vi "run.vi"(8 "error in (no error)":errorcluster, 11 "IntrinsicImagingMG091001 in":refnum<class "DataCollectionMG091001IntrinsicImaging.lvclass">) -> (0 "error out":errorcluster, 3 "IntrinsicImagingMG091001 out":refnum<class "DataCollectionMG091001IntrinsicImaging.lvclass">)   [LabVIEW 2010, in "DataCollectionMG091001IntrinsicImaging.lvclass"]
uses:
  DataCollectionMG091001IntrinsicImaging.lvclass
  sweep_part_enum.ctl
  average_save_type_enum.ctl
  individual_sweeps_saving_enum.ctl
  main/labview_source/controls/undock_button.ctl
  DataCollectionMG091001IntrinsicImaging.lvclass/DataCollectionMG091001IntrinsicImaging.ctl
  DataCollectionDL091104Scaffold/DataCollectionDL091104Scaffold/DataCollectionDL091104Scaffold.lvclass
  common/classes/ErrorController/ErrorController/class_data.vi
  GenericDataCollection/GenericDataCollection/GenericDataCollection.lvclass
  common/classes/ErrorController/ErrorController/ErrorController.lvclass
panel:
  in  "button:undock":T1
  in  "Tab Control":enum32{"User", "About"}(tab)
  in  "Sweep":i32(slide) scale=1.0..1.1
  in  "average over time":bool
  in  "Average over sweeps?":bool
  in  "average save type enum":T2 caption="What to save..."
  in  "include sweep?":bool
  in  "Time":dbl[unit](slide) min=0.0 scale=0.0..1.0
  in  "sweep part":T3
  in  "overlay button":bool
  in  "save control?":bool
  in  "How to save individual sweeps:":T4
  in  "finished?":bool
  # "Browse data"
  # "Saving parameters"
  # "DataCollectionMG091001IntrinsicImaging\n\nImplemented by:\nMaurice Göldi, University of Zürich, Switezrland"
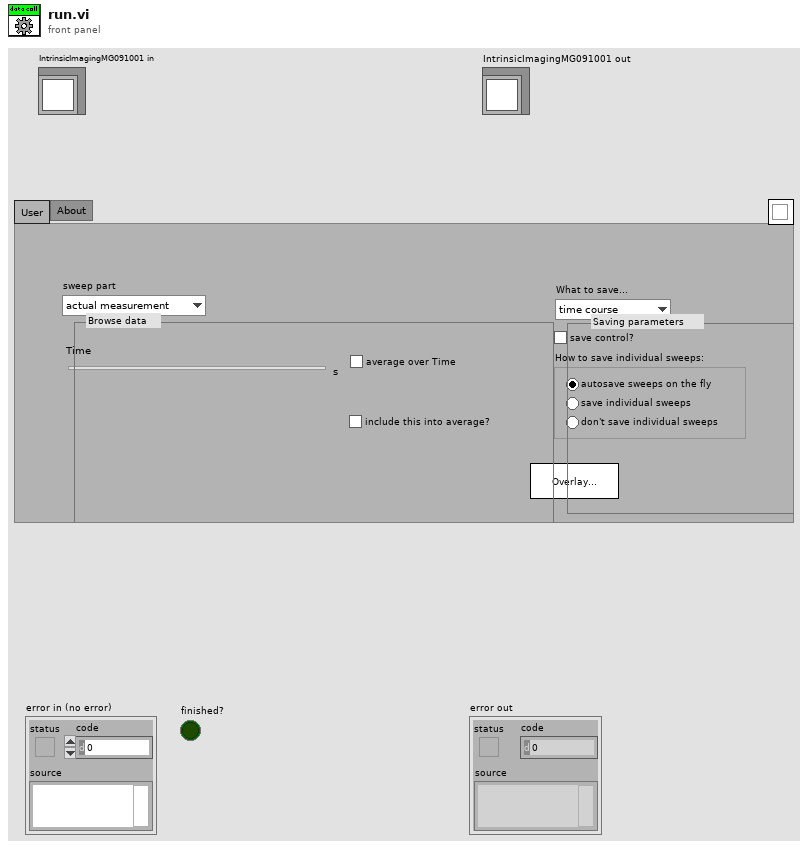
[diagram p1: front panel]
types:
  T1 = typedef "undock_button.ctl" = bool
  T2 = typedef "DataCollectionMG091001IntrinsicImaging.lvclass/average_save_type_enum.ctl" = enum16{"time course", "time average", "time course and average"}
  T3 = typedef "DataCollectionMG091001IntrinsicImaging.lvclass/sweep_part_enum.ctl" = enum16{"actual measurement", "control"}
  T4 = typedef "DataCollectionMG091001IntrinsicImaging.lvclass/individual_sweeps_saving_enum.ctl" = enum32{"autosave sweeps on the fly", "save individual sweeps", "don't save individual sweeps"}
  T5 = enum8{"Enabled", "Disabled", "Disabled and Grayed Out"}
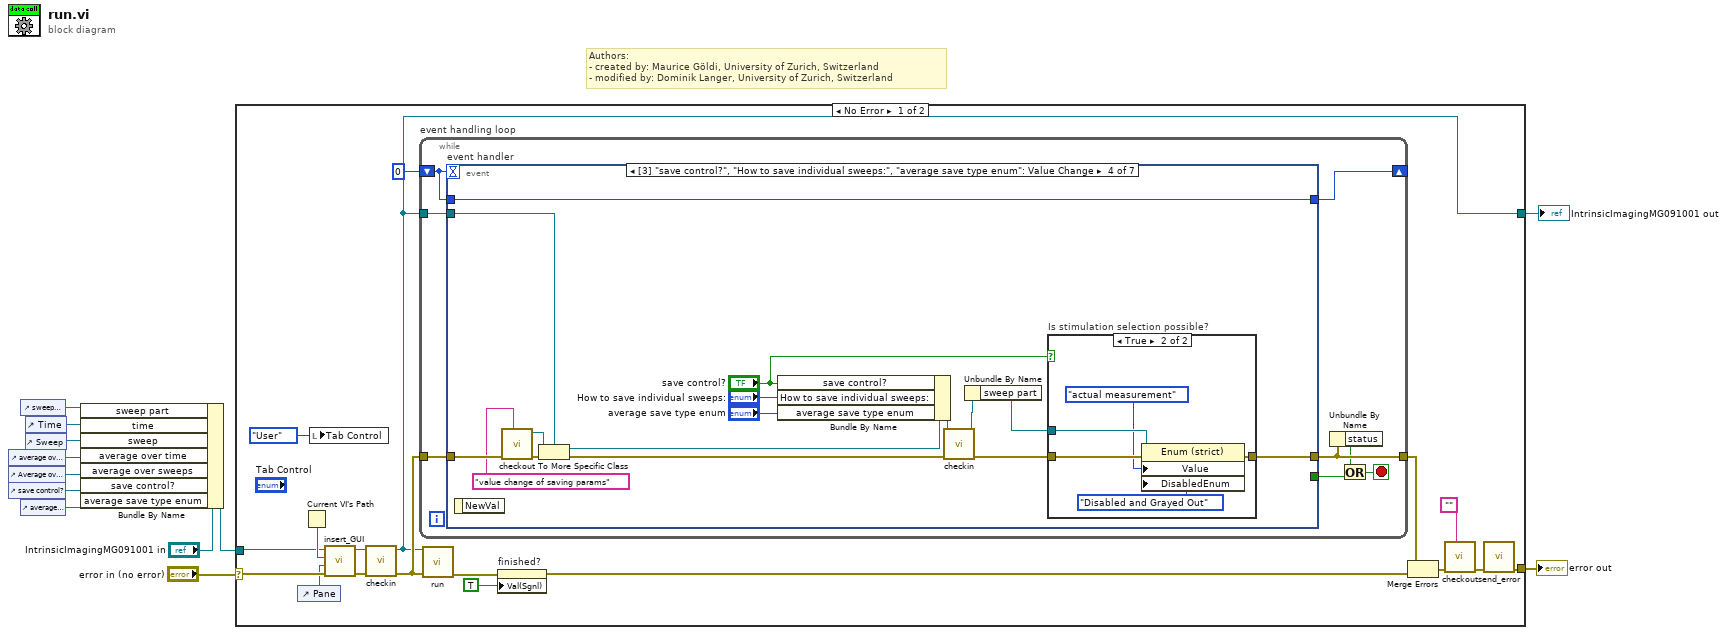
[diagram p0: block diagram]
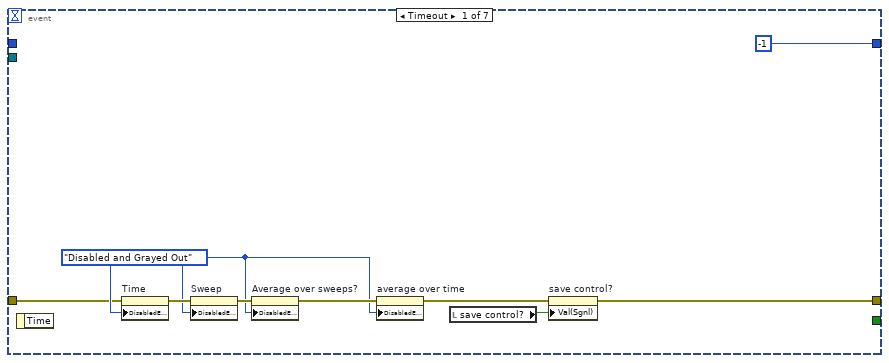
[diagram p2: hidden frame]
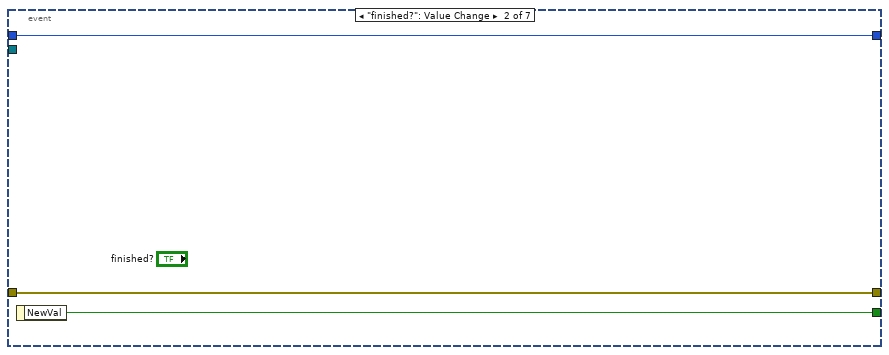
[diagram p3: hidden frame]
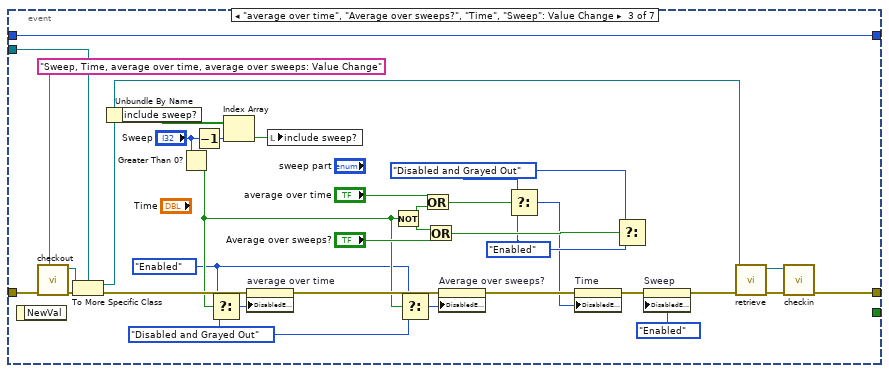
[diagram p4: hidden frame]
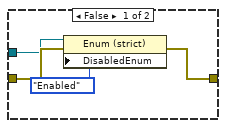
[diagram p5: hidden frame]
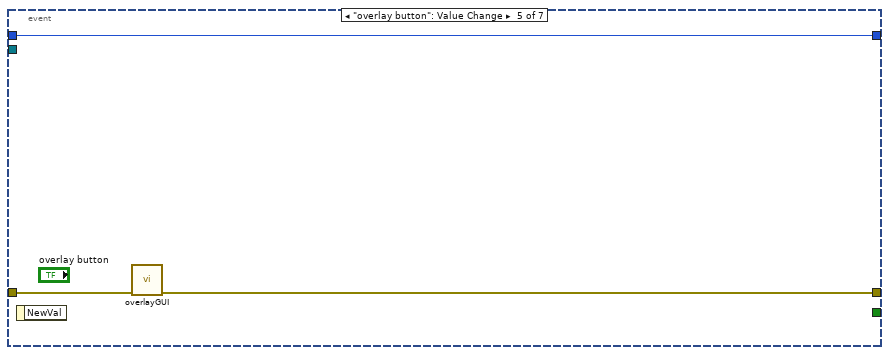
[diagram p6: hidden frame]
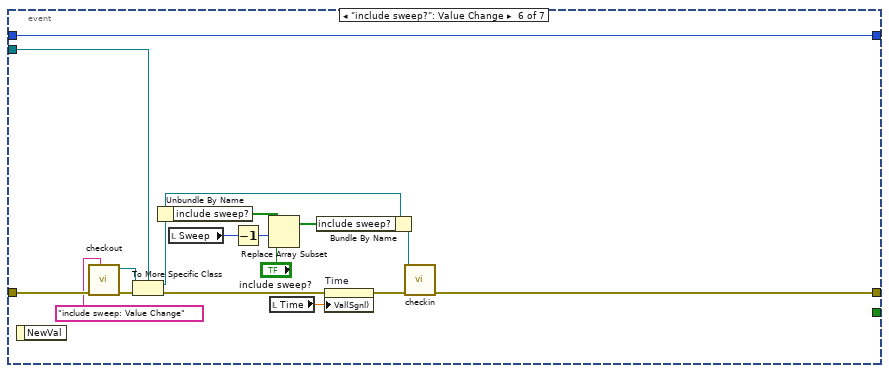
[diagram p7: hidden frame]
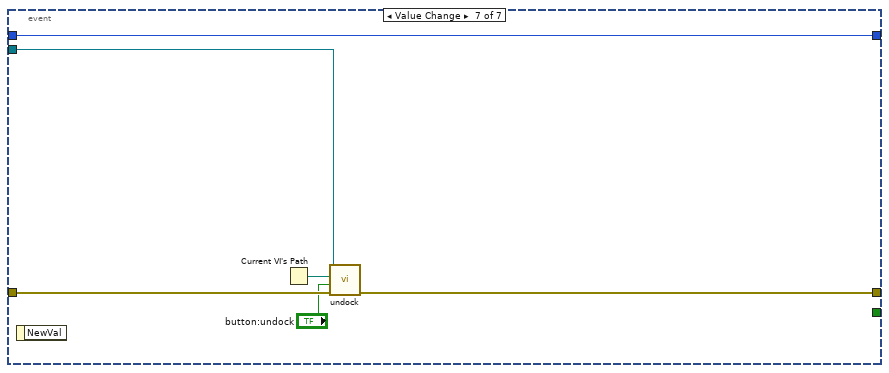
[diagram p8: hidden frame]
diagram:
  # "Authors: \n- created by: Maurice Göldi, University of Zurich, Switzerland\n- modified by: Dominik Langer, University of Zurich, Switzerland"
  n1 = control-ref of="average over time"() -> (w7:refnum<vi>)
  n2 = control-ref of="Average over sweeps?"() -> (w8:refnum<vi>)
  n3 = control-ref of="save control?"() -> (w4:refnum<vi>)
  n4 = control-ref of="sweep part"() -> (w1:refnum<vi>)
  n5 = control-ref of="average save type enum"() -> (w3:refnum<vi>)
  n6 = control-ref of="Time"() -> (w2:refnum<vi>)
  n7 = control-ref of="Sweep"() -> (w9:refnum<vi>)
  n8 = Bundle By Name(cluster="IntrinsicImagingMG091001 in", "sweep part"=w1, "time"=w2, "sweep"=w9, "average over time"=w7, "average over sweeps"=w8, "save control?"=w4, "average save type enum"=w3) -> (w5:refnum<class "DataCollectionMG091001IntrinsicImaging.lvclass">)
  n9 = case shown="No Error" "error in (no error)" {
    selector: "error in (no error)" -> [w21 w135]
    tunnel: [w17 w135] -> w12
    tunnel: [w15 w136] -> w11
    tunnel: w5 -> [w20 w136]
    frame No Error {
      n10 = control-ref of="Pane"() -> (w19:refnum<vi>)
      n11 = Current VI's Path() -> (path=w22:path)
      n12 = local write "Tab Control"(enum32{"User", "About"}."User" ("Tab Control")) -> ()
      n13 = call-dynamic "insert_GUI.vi"("error in (no error)"=w21, "Pane"=w19, "VI path"=w22, "GenericComponent in"=w20) -> ("error out"=w13:errorcluster, "GenericComponent out"=w14:refnum<class "DataCollectionMG091001IntrinsicImaging.lvclass">)  [unwired: 6 in]
      n14 = call-dynamic "checkin.vi"("error in (no error)"=w13, "GenericDataCollection in"=w14) -> ("error out"=w27:errorcluster, "GenericDataCollection out"=w15:refnum<class "DataCollectionMG091001IntrinsicImaging.lvclass">)  [unwired: 8 in]
      n15 = while "event handling loop" {
        shift-right: [w36] -> _
        shift-left: 0 -> [w35]
        tunnel: w27 -> [w38]
        tunnel: [w33] -> w26
        tunnel: w15 -> [w37]
        stop <- w31 stop-if-true
        n16 = event "event handler" shown="[3] \"save control?\", \"How to save individual sweeps:\", \"average save type enum\": Value Change" {
          selector: _ -> [_ _ _ _ _ _ _]
          dyn-events: _ -> [_ _ _ _ _ _ _]
          timeout: w35 -> [_ _ _ _ _ _ _]
          tunnel: [w40 w49 w81 w87 w109 w112 w131] -> w33
          tunnel: w38 -> [w39 w49 w82 w95 w110 w117 w132]
          tunnel: w37 -> [_ _ w78 w96 _ w120 w133]
          tunnel: [-1 w50 w83 w99 w111 w128 w134] -> w36
          tunnel: w35 -> [_ w50 w83 w99 w111 w128 w134]
          tunnel: [_ w48 _ _ _ _ _] -> w34
          event Timeout {
            w43 = T5."Disabled and Grayed Out" ("Disabled")
            n17 = event-data() -> ()  [unwired: 1 in, 1 out]
            n18 = property on="Time" class="Slide (strict)"(error in=w39, "DisabledEnum"=w43) -> (error out=w44:errorcluster)  [unwired: 1 in, 1 out]
            n19 = property on="Sweep" class="Slide (strict)"(error in=w44, "DisabledEnum"=w43) -> (error out=w45:errorcluster)  [unwired: 1 in, 1 out]
            n20 = property on="Average over sweeps?" class="Bool (strict)"(error in=w45, "DisabledEnum"=w43) -> (error out=w46:errorcluster)  [unwired: 1 in, 1 out]
            n21 = property on="average over time" class="Bool (strict)"(error in=w46, "DisabledEnum"=w43) -> (error out=w41:errorcluster)  [unwired: 1 in, 1 out]
            n22 = local read "save control?"() -> (w42:bool)
            n23 = property on="save control?" class="Bool (strict)"(error in=w41, "Val(Sgnl)"=w42) -> (error out=w40:errorcluster)  [unwired: 1 in, 1 out]
          }
          event "finished?": Value Change {
            n24 = event-data() -> ("NewVal"=w48:bool)  [unwired: 1 in]
          }
          event "average over time", "Average over sweeps?", "Time", "Sweep": Value Change {
            w59 = T5."Disabled and Grayed Out" ("Disabled")
            w58 = T5."Enabled" ("Disabled")
            w62 = T5."Disabled and Grayed Out" ("f")
            w61 = T5."Enabled" ("Disabled")
            n25 = event-data() -> ()  [unwired: 1 in, 1 out]
            n26 = call "checkout.vi"("locked by?"="Sweep, Time, average over time, average over sweeps: Value Change", "error in (no error)"=w82) -> ("error out"=w80:errorcluster, "GenericDataCollection out"=w79:refnum<class "GenericDataCollection.lvclass">)  [unwired: 8 in]
            n27 = To More Specific Class(target class=w78, reference=w79, error in=w80) -> (specific class reference=w52:refnum<class "DataCollectionMG091001IntrinsicImaging.lvclass">, error out=w68:errorcluster)
            n28 = Unbundle By Name(w52) -> ("include sweep?"=w76:bool[])
            n29 = Greater Than 0?(x="Sweep") -> (x > 0?=w64:bool)
            n30 = Decrement(x="Sweep") -> (x-1=w74:i32)
            n31 = Select(t=w61, s=w64, f=w62) -> (s? t:f=w67:T5)
            n32 = Index Array(array=w76, index=w74) -> (element=w75:bool)
            n33 = property on="average over time" class="Bool (strict)"(error in=w68, "DisabledEnum"=w67) -> (error out=w72:errorcluster)  [unwired: 1 in, 1 out]
            n34 = local write "include sweep?"(w75) -> ()
            n35 = Not(x=w64) -> (.not. x?=w70:bool)
            n36 = Select(t=w61, s=w64, f=w62) -> (s? t:f=w63:T5)
            n37 = Or(x="average over time", y=w70) -> (x .or. y?=w60:bool)
            n38 = Or(x=w70, y="Average over sweeps?") -> (x .or. y?=w65:bool)
            n39 = property on="Average over sweeps?" class="Bool (strict)"(error in=w72, "DisabledEnum"=w63) -> (error out=w69:errorcluster)  [unwired: 1 in, 1 out]
            n40 = Select(t=w59, s=w60, f=w58) -> (s? t:f=w57:T5)
            n41 = property on="Time" class="Slide (strict)"(error in=w69, "DisabledEnum"=w57) -> (error out=w55:errorcluster)  [unwired: 1 in, 1 out]
            n42 = Select(t=w59, s=w65, f=w58) -> ()  [unwired: 1 out]
            n43 = property on="Sweep" class="Slide (strict)"(error in=w55, "DisabledEnum"=T5."Enabled" ("Disabled")) -> (error out=w54:errorcluster)  [unwired: 1 in, 1 out]
            n44 = call-dynamic "retrieve.vi"("error in (no error)"=w54, "DL090215DataCollection in"=w52) -> ("error out"=w53:errorcluster, "DL090215DataCollection out"=w51:refnum<class "DataCollectionMG091001IntrinsicImaging.lvclass">)  [unwired: 8 in]
            n45 = call-dynamic "checkin.vi"("error in (no error)"=w53, "GenericDataCollection in"=w51) -> ("error out"=w81:errorcluster)  [unwired: 8 in, 1 out]
          }
          event "save control?": Value Change {
            n46 = event-data() -> ()  [unwired: 1 in, 1 out]
            n47 = call "checkout.vi"("locked by?"="value change of saving params", "error in (no error)"=w95) -> ("error out"=w94:errorcluster, "GenericDataCollection out"=w93:refnum<class "GenericDataCollection.lvclass">)  [unwired: 8 in]
            n48 = To More Specific Class(target class=w96, reference=w93, error in=w94) -> (specific class reference=w92:refnum<class "DataCollectionMG091001IntrinsicImaging.lvclass">, error out=w90:errorcluster)
            n49 = Bundle By Name(cluster=w92, "save control?"="save control?", "How to save individual sweeps:"="How to save individual sweeps:", "average save type enum"="average save type enum") -> (w91:refnum<class "DataCollectionMG091001IntrinsicImaging.lvclass">)
            n50 = call-dynamic "checkin.vi"("error in (no error)"=w90, "GenericDataCollection in"=w91) -> ("error out"=w88:errorcluster, "GenericDataCollection out"=w86:refnum<class "DataCollectionMG091001IntrinsicImaging.lvclass">)  [unwired: 8 in]
            n51 = Unbundle By Name(w86) -> ("sweep part"=w85:refnum<vi>)
            n52 = case "Is stimulation selection possible?" shown="True" "save control?" {
              tunnel: w88 -> [w103 w108]
              tunnel: [w102 w107] -> w87
              tunnel: w85 -> [w101 w106]
              frame False {
                n53 = property class="Enum (strict)"(reference=w101, error in=w103, "DisabledEnum"=T5."Enabled" ("Disabled")) -> (error out=w102:errorcluster)  [unwired: 1 out]
              }
              frame True {
                n54 = property class="Enum (strict)"(reference=w106, error in=w108, "Value"=enum16{"actual measurement", "control"}."actual measurement", "DisabledEnum"=T5."Disabled and Grayed Out" ("Disabled")) -> (error out=w107:errorcluster)  [unwired: 1 out]
              }
            }
          }
          event "overlay button": Value Change {
            n55 = event-data() -> ()  [unwired: 1 in, 1 out]
            n56 = call "overlayGUI.vi"("error in (no error)"=w110) -> ("error out"=w109:errorcluster)  [unwired: 10 in]
          }
          event "include sweep?": Value Change {
            n57 = event-data() -> ()  [unwired: 1 in, 1 out]
            n58 = call "checkout.vi"("locked by?"="include sweep: Value Change", "error in (no error)"=w117) -> ("error out"=w122:errorcluster, "GenericDataCollection out"=w121:refnum<class "GenericDataCollection.lvclass">)  [unwired: 8 in]
            n59 = To More Specific Class(target class=w120, reference=w121, error in=w122) -> (specific class reference=w119:refnum<class "DataCollectionMG091001IntrinsicImaging.lvclass">, error out=w114:errorcluster)
            n60 = Unbundle By Name(w119) -> ("include sweep?"=w126:bool[])
            n61 = local read "Sweep"() -> (w123:i32)
            n62 = Decrement(x=w123) -> (x-1=w124:i32)
            n63 = Replace Array Subset(array=w126, new element="include sweep?", index=w124) -> (w125:bool[])
            n64 = local read "Time"() -> (w115:dbl[unit])
            n65 = Bundle By Name(cluster=w119, "include sweep?"=w125) -> (w118:refnum<class "DataCollectionMG091001IntrinsicImaging.lvclass">)
            n66 = property on="Time" class="Slide (strict)"(error in=w114, "Val(Sgnl)"=w115) -> (error out=w113:errorcluster)  [unwired: 1 in, 1 out]
            n67 = call-dynamic "checkin.vi"("error in (no error)"=w113, "GenericDataCollection in"=w118) -> ("error out"=w112:errorcluster)  [unwired: 8 in, 1 out]
          }
          event Value Change {
            n68 = event-data() -> ()  [unwired: 1 in, 1 out]
            n69 = Current VI's Path() -> (path=w129:path)
            n70 = call-dynamic "undock.vi"("error in (no error)"=w132, "undock?"="button:undock", "VI path"=w129, "GenericComponent in"=w133) -> ("error out"=w131:errorcluster)  [unwired: 6 in, 1 out]
          }
        }
        n71 = Unbundle By Name(w33) -> ("status"=w32:bool)
        n72 = Or(x=w32, y=w34) -> (x .or. y?=w31:bool)
      }
      n73 = call-parent "run.vi"("error in (no error)"=w27, "DataCollectionDL091104Scaffold.lvclass out"=w15) -> ("error out"=w30:errorcluster)  [unwired: 8 in, 1 out]
      n74 = property on="finished?" class="Bool (strict)"(error in=w30, "Val(Sgnl)"=TRUE ("Value (Signaling)")) -> (error out=w29:errorcluster)  [unwired: 1 in, 1 out]
      n75 = Merge Errors(w26, w29) -> (w24:errorcluster)
      n76 = call "checkout.vi"("locked by?"="", "error in (no error)"=w24) -> ("error out"=w18:errorcluster)  [unwired: 8 in, 1 out]
      n77 = call "send_error.vi"("error in (no error)"=w18) -> ("error out"=w17:errorcluster)  [unwired: 10 in]
    }
    frame Error {
    }
  }
  "error out" <- w12
  "IntrinsicImagingMG091001 out" <- w11
